vi "datasourceConfigs.to_json.vi"(8 "error in":errorcluster, 10 "datasourceConfigs":T1[](array[typedef])) -> (0 "error out":errorcluster, 2 "json":string)   [LabVIEW 2020, in "type.lvclass"]
uses:
  type.lvclass
  datasourceConfig.ctl
  7a922176-cc80-476e-b002-4975f22ae696.vi
  <vilib>/JDP Science/JSONtext/Variant to JSON Text.vi
  <vilib>/JDP Science/JSONtext/LVClass Serializer/JSONtext LVClass Serializer.lvclass
  type.lvclass/type.ctl
  <vilib>/JDP Science/JSONtext/JSONtext.lvlib
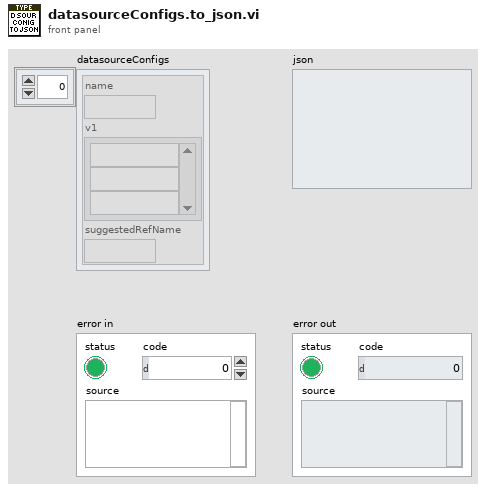
[diagram p1: front panel]
types:
  T1 = typedef "type.lvclass/datasourceConfig.ctl" = cluster{"name":string, "v1":string[], "suggestedRefName":string}
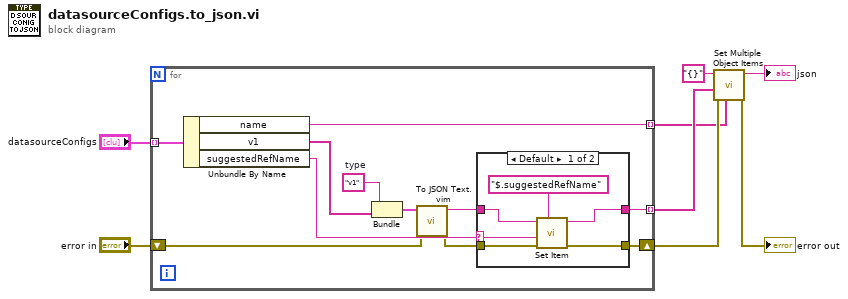
[diagram p0: block diagram]
diagram:
  n1 = for {
    tunnel: "datasourceConfigs" -> [w19] mode=indexing
    tunnel: [w18] -> w2 mode=indexing
    tunnel: [w13] -> w7 mode=indexing
    shift-right: [w10] -> w5
    shift-left: "error in" -> [w9]
    w17 = "v1"  # type
    n2 = Unbundle By Name(w19) -> ("name"=w18:string, "v1"=w16:string[], "suggestedRefName"=w14:string)
    n3 = Bundle("type"=w17, "v1"=w16) -> (w15:cluster{"type":string, "v1":string[]})  [unwired: 1 in]
    n4 = call "To JSON Text.vim"("error in (no error)"=w9, "Anything"=w15) -> ("error out"=w11:errorcluster, "<JSON>"=w12:string)  [unwired: 8 in]
    n5 = case shown="Default" w14 {
      selector: w14 -> [w24 _]
      tunnel: [w23 w27] -> w13
      tunnel: w12 -> [w25 w27]
      tunnel: w11 -> [w21 w26]
      tunnel: [w20 w26] -> w10
      frame Default {
        n6 = call <vilib>:"Set Item.vi"("$Path or Item Name"="$.suggestedRefName", "error in (no error)"=w21, "JSON to Insert"=w24, "JSON"=w25) -> ("error out"=w20:errorcluster, "<JSON>"=w23:string)  [unwired: 4 in, 1 out]
      }
      frame "" {
      }
    }
  }
  n7 = call <vilib>:"Set Multiple Object Items.vi"("Item Names"=w2, "error in (no error)"=w5, "JSON Items"=w7, "JSON"="{}") -> ("error out"=→"error out":errorcluster, "<JSON>"=→"json":string)  [unwired: 5 in]
